vi "LIA Debugging Host.vi"() -> ()   [LabVIEW 2017]
uses:
  Program Files (x86)/National Instruments/LabVIEW 2017/examples/Lock-In Amplifier/lib/host/Public/pll settings.ctl
  Program Files (x86)/National Instruments/LabVIEW 2017/examples/Lock-In Amplifier/lib/host/Public/lock-in settings.ctl
  Program Files (x86)/National Instruments/LabVIEW 2017/examples/Lock-In Amplifier/lib/interface/Interface FPGA/LIA Host Interface FPGA.lvclass
  C:/Program Files (x86)/National Instruments/LabVIEW 2017/examples/Lock-In Amplifier/lib/interface/Interface/LIA Host Interface.lvclass
  Program Files (x86)/National Instruments/LabVIEW 2017/examples/Lock-In Amplifier/lib/host/Public/fpga type.ctl
  <vilib>/Analysis/4window.llb/windowTd.ctl
  <vilib>/measure/maspectr.llb/FFT Spectrum (Mag-Phase) for N Chan.vi
  Program Files (x86)/National Instruments/LabVIEW 2017/examples/Lock-In Amplifier/lib/interface/Interface FPGA/Properties/FpgaSession_GET.vi
  <vilib>/Utility/error.llb/Error Cluster From Error Code.vi
  <vilib>/rvi/errors/niLvFpgaAdjustHostInterfaceError.vi
  <vilib>/measure/maspectr.llb/FFT Power Spectrum and PSD for 1 Chan (CDB).vi
  <vilib>/measure/maspectr.llb/FFT Power Spectrum and PSD for N Chan.vi
  <vilib>/rvi/interface/nirviReadWriteControl/nirviReadWriteControl.xnode
  Program Files (x86)/National Instruments/LabVIEW 2017/examples/Lock-In Amplifier/lib/interface/Interface/LIA Host Interface.lvclass
  Program Files (x86)/National Instruments/LabVIEW 2017/examples/Lock-In Amplifier/lib/host/Lock-In Amplifier Example Host.lvlib
  Program Files (x86)/National Instruments/LabVIEW 2017/examples/Lock-In Amplifier/lib/shared/Lock-In Amplifier Example Shared.lvlib
  <vilib>/measure/NI_MAPro.lvlib
  NiFpgaLv.dll
  <vilib>/rvi/interface/Simulation/niFpgaSimulationCallBeginRW.vi
  <vilib>/Analysis/NI_AALPro.lvlib
  <vilib>/Analysis/NI_AALBase.lvlib
  <vilib>/ptbypt/NI_PtbyPt.lvlib
panel:
  in  "Tab Control 2":enum32{"Page 1", "Page 2"}(tab)
  in  "dpll.m 0":i8=-20
  in  "averaging lia":T1={"averaging mode"=enum."RMS averaging", "weighting mode"=enum."Exponential", "number of averages"=10}
  in  "restart averaging  lia":bool
  in  "lock-in.decimator0 0":enum16{"None", "CIC", "FIR", "4HB"}(ring)=enum."FIR"
  in  "lock-in.decimator1 0":enum16{"None", "FIR"}(ring)
  in  "averaging preview":T1={"averaging mode"=enum."RMS averaging", "weighting mode"=enum."Exponential", "number of averages"=10}
  in  "restart averaging preview":bool
  out "lock-in.max-min":dbl=1.9775797561733533e-07 caption="Deviation" format="%#_6p"
  out "lock-in.min":dbl=1.9775797561733533e-07 caption="Deviation" format="%#_6p"
  out "lock-in.max":dbl=1.9775797561733533e-07 caption="Deviation" format="%#_6p"
  in  "Tab Control 1":T2(tab)
  out "pll.vco output 0":fxp<+/-,48,0> format="%#.18g"
  out "lock-in.cic config 0":cluster{"factor":fxp<+,16,16>, "shift":i16}
  out "dpll.vco output 0":fxp<+/-,48,0> format="%#.18g"
  out "dpll.config 0":T3
  out "nco.frequency 0":fxp<+/-,48,0>=0.0010000000000012221 format="%#_48g"
  out "Waveform Graph 5":cluster{"f0":dbl, "df":dbl, "magnitude":dbl[]}(graph)
  out "Waveform Graph 2":cluster{"f0":dbl, "df":dbl, "magnitude":dbl[]}[](graph)
  out "Waveform Graph 3":dbl[][](graph)
  out "Waveform Graph 4":dbl[][](graph)
  out "Waveform Graph":cluster{"f0":dbl, "df":dbl, "magnitude":dbl[]}[](graph)
  in  "app.quit":bool
  in  "lock-in.record length 0":u32=2048 caption="Record Length"
  in  "app.tab 0":enum32{"Lock-In", "PLL"}(tab)
  in  "lock-in.decimation1 0":i32=2048 caption="Decimation 1"
  in  "lock-in.sampling rate":dbl=100000000.0 caption="Sampling Rate" format="%_10p"
  in  "lock-in.decimation0 0":i32=2048 caption="Decimation 0"
  in  "lock-in.source 0":enum16{"AI 0", "AI 1", "AI 2", "AI 3", "NCO 0"}(ring)=enum."AI 1" caption="Channel"
  in  "lock-in.carrier 0":T4(ring)=enum."DPLL 0" caption="Carrier Source"
  in  "lock-in.manual carrier 0":dbl=100000.0 caption="Carrier Frequency" format="%_10p"
  in  "pll.source 0":enum16{"AI 0", "AI 1", "AI 2", "AI 3"}(ring) caption="Source"
  in  "pll.q frequency 0":dbl=100000.0 caption="Q Frequency" format="%#_6p"
  in  "pll.reset 0":bool caption="PLL Reset"
  in  "rio device":tag="PXI1Slot8" caption="Resource"
  out "lock-in.deviation":dbl=1.9775797561733533e-07 caption="Deviation" format="%#_6p"
  out "lock-in.amplitude":dbl=8.221341747482856e-05 caption="lock-in.mean" format="%#_12p"
  out "Result":cluster{dbl, "standard deviation":dbl}(graph)
  # "NI Lock-In Amplifier Reference Example"
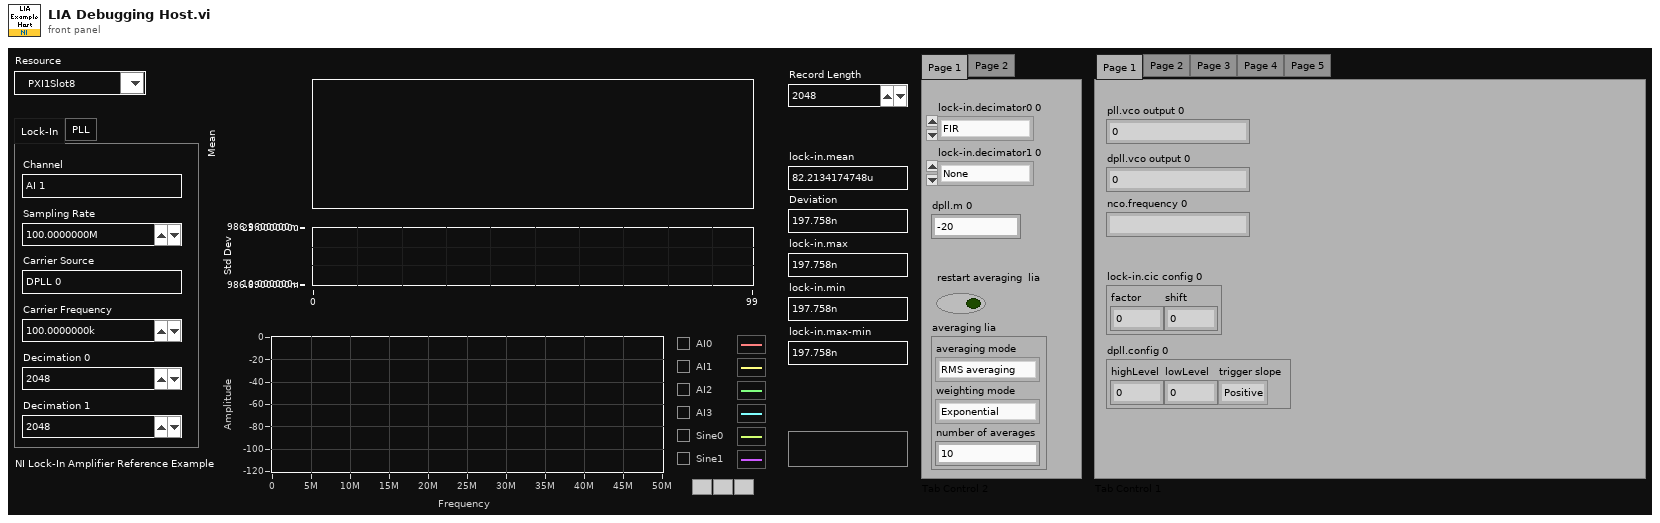
[diagram p1: front panel]
types:
  T1 = cluster{"averaging mode":enum16{"No averaging", "Vector averaging", "RMS averaging", "Peak hold"}, "weighting mode":enum16{"Linear", "Exponential"}, "number of averages":u32}
  T2 = enum32{"Page 1", "Page 2", "Page 3", "Page 4", "Page 5"}
  T3 = cluster{"highLevel":fxp<+/-,18,1>, "lowLevel":fxp<+/-,18,1>, "trigger slope":enum8{"Positive", "Negative"}}
  T4 = enum16{"Manual 0", "Manual 1", "Manual 2", "Manual 3", "PLL 0", "PLL 1", "DPLL 0", "DPLL 1"}
  T5 = typedef "Lock-In Amplifier Example Host.lvlib/lock-in settings.ctl" = cluster{"decimation":i32, "source":i32, "carrier source":i32, "carrier":dbl}
  T6 = typedef "Lock-In Amplifier Example Host.lvlib/pll settings.ctl" = cluster{"source":i32, "q frequency":dbl}
  T7 = typedef "NI_AALPro.lvlib/windowTd.ctl" = u32
  T8 = cluster{"dB On (F)":bool, "unwrap phase (F)":bool, "convert to degree (F)":bool}
  T9 = typedef "Lock-In Amplifier Example Host.lvlib/fpga type.ctl" = refnum<k20>
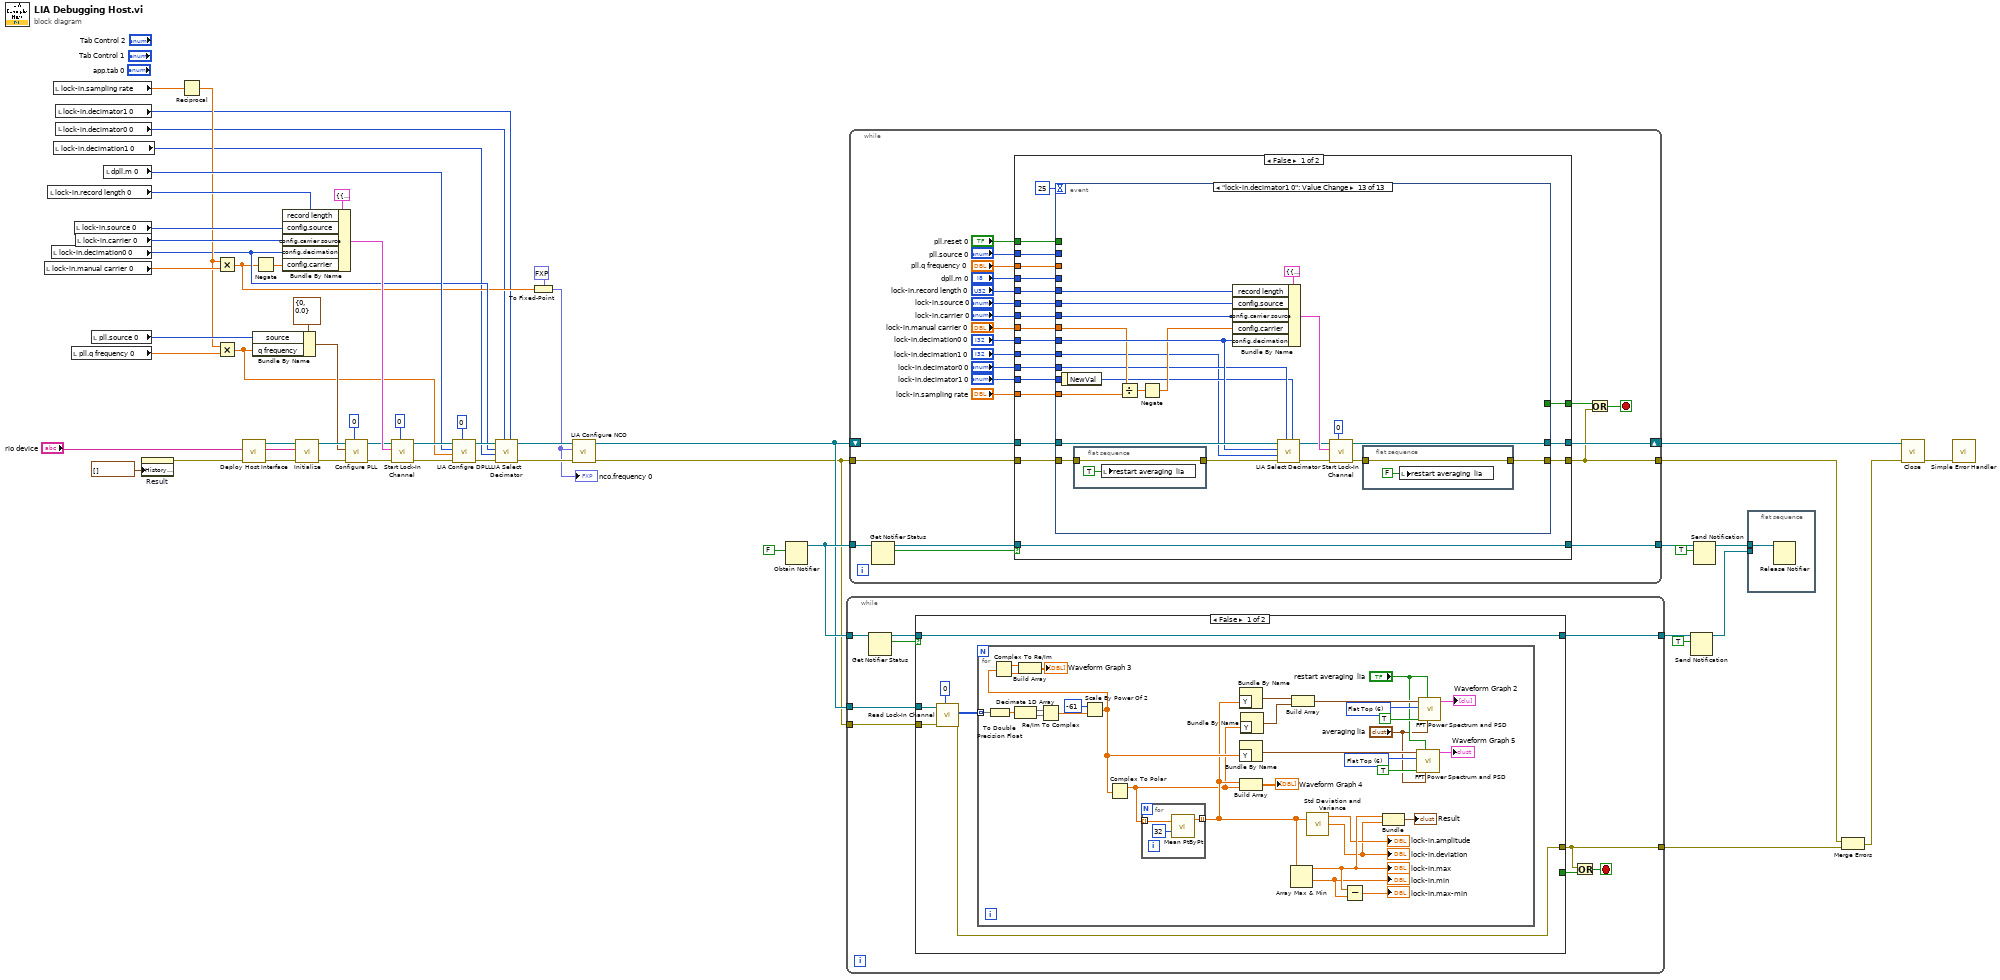
[diagram p0: block diagram]
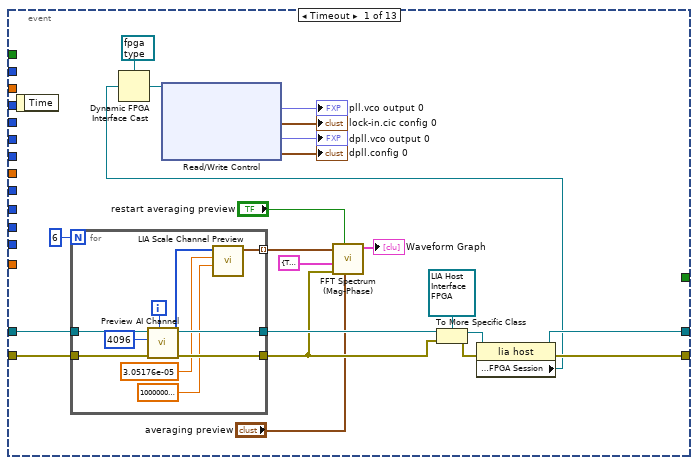
[diagram p2: hidden frame]
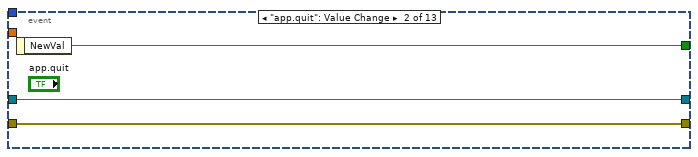
[diagram p3: hidden frame]
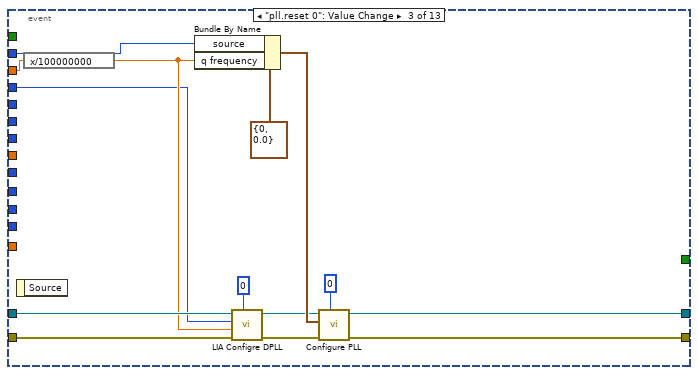
[diagram p4: hidden frame]
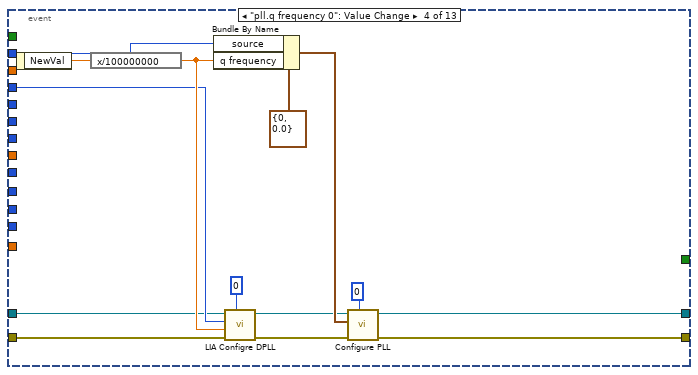
[diagram p5: hidden frame]
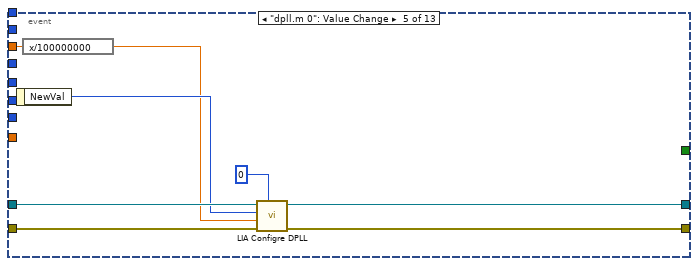
[diagram p6: hidden frame]
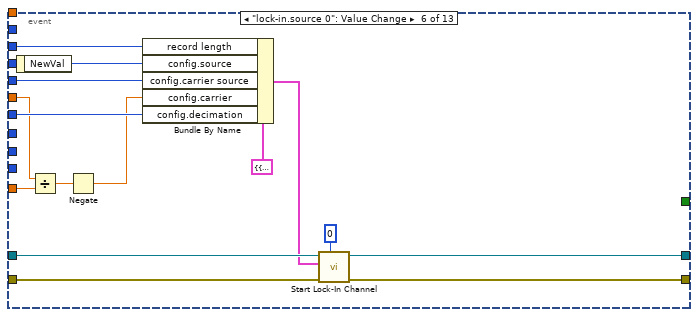
[diagram p7: hidden frame]
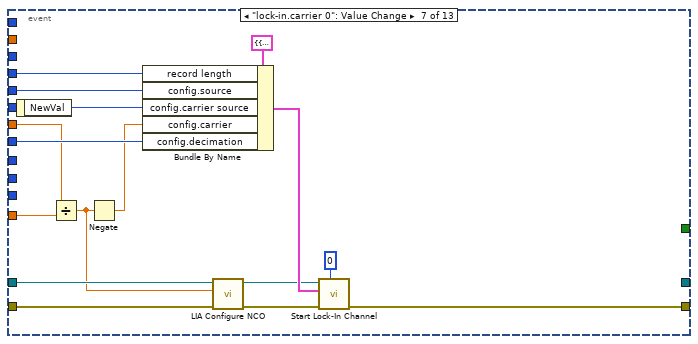
[diagram p8: hidden frame]
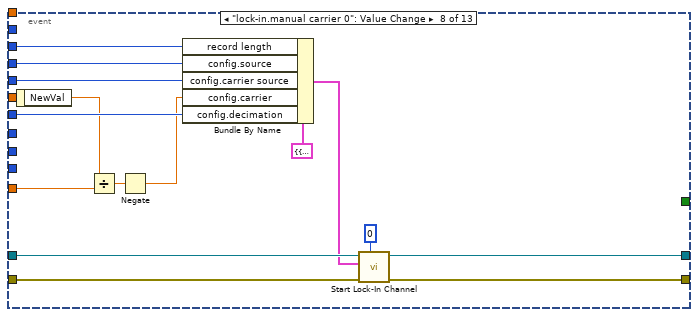
[diagram p9: hidden frame]
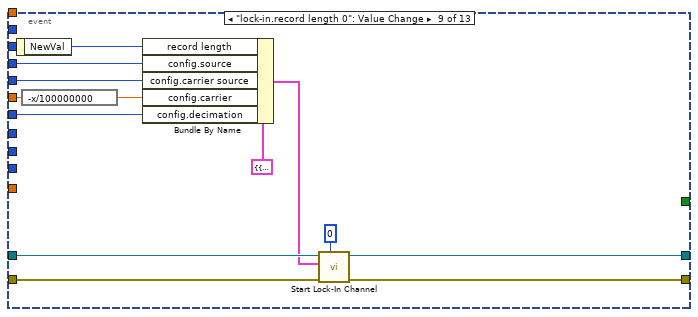
[diagram p10: hidden frame]
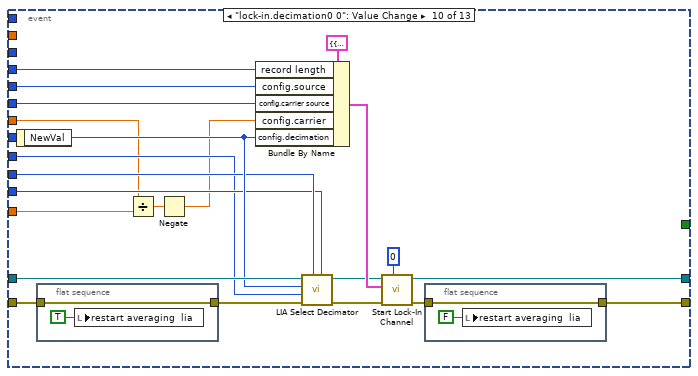
[diagram p11: hidden frame]
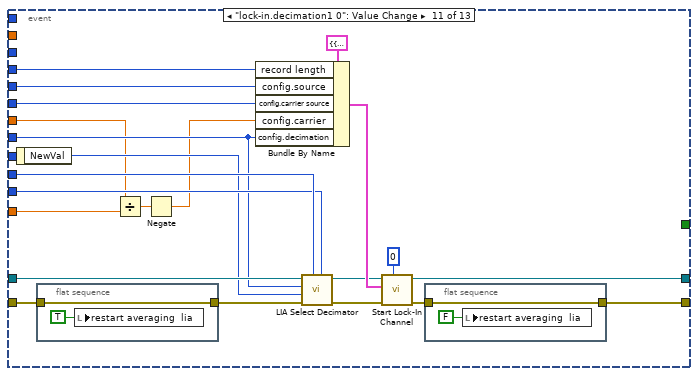
[diagram p12: hidden frame]
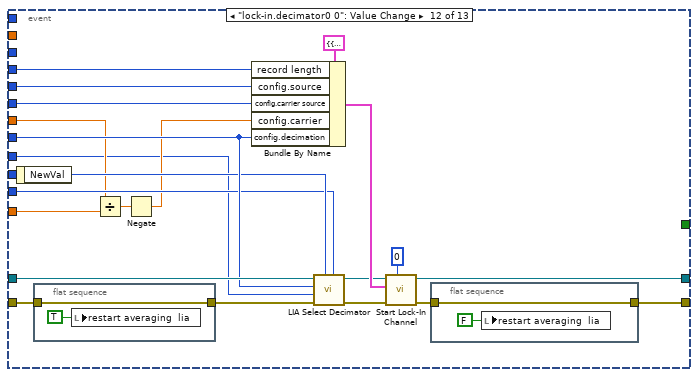
[diagram p13: hidden frame]
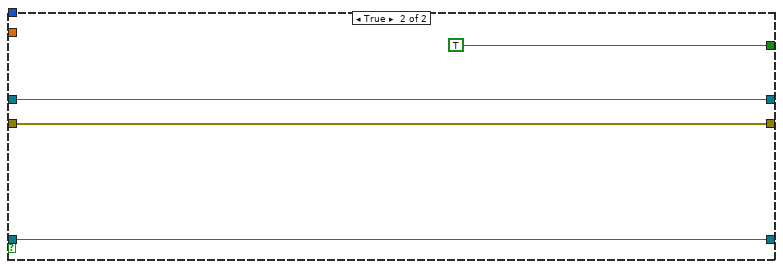
[diagram p14: hidden frame]
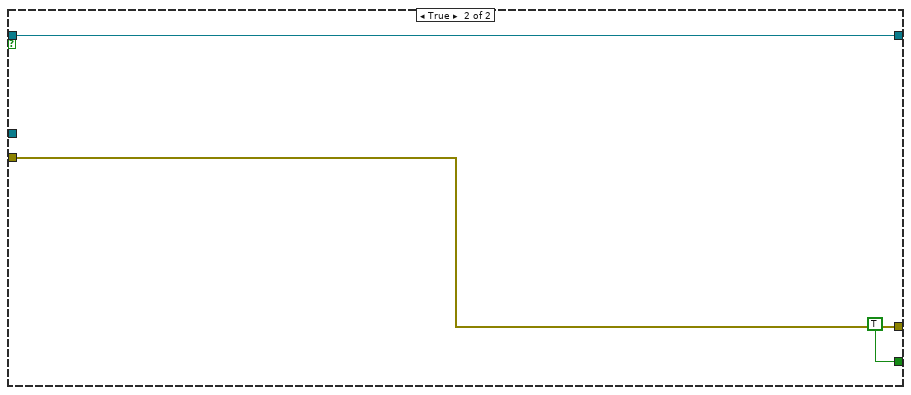
[diagram p15: hidden frame]
diagram:
  n1 = local read "lock-in.manual carrier 0"() -> (w51:dbl)
  n2 = local read "lock-in.record length 0"() -> (w32:u32)
  n3 = local read "lock-in.decimation0 0"() -> (w7:i32)
  n4 = local read "lock-in.sampling rate"() -> (w8:dbl)
  n5 = local read "lock-in.decimation1 0"() -> (w1:i32)
  n6 = local read "lock-in.decimator1 0"() -> (w2:enum16{"None", "FIR"})
  n7 = local read "lock-in.decimator0 0"() -> (w3:enum16{"None", "CIC", "FIR", "4HB"})
  n8 = local read "pll.q frequency 0"() -> (w52:dbl)
  n9 = local read "lock-in.source 0"() -> (w56:enum16{"AI 0", "AI 1", "AI 2", "AI 3", "NCO 0"})
  n10 = local read "lock-in.carrier 0"() -> (w55:T4)
  n11 = local read "pll.source 0"() -> (w53:enum16{"AI 0", "AI 1", "AI 2", "AI 3"})
  n12 = local read "dpll.m 0"() -> (w18:i8)
  n13 = property on="Result" class="WFChart (strict)"("History Data"=cluster{dbl, "standard deviation":dbl}[] []) -> (error out=w27:errorcluster)  [unwired: 2 in, 1 out]
  n14 = Reciprocal(x=w8) -> (1/x=w13:dbl)
  n15 = Multiply(x=w13, y=w51) -> (x*y=w6:dbl)
  n16 = Multiply(x=w13, y=w52) -> (x*y=w11:dbl)
  n17 = call "Deploy Host Interface.vi"("error in"=w27, "resource"="rio device") -> ("error out"=w28:errorcluster, "resource out"=w29:string, "lia host interface"=w30:refnum<class "LIA Host Interface.lvclass">)  [unwired: 7 in]
  n18 = Bundle By Name(cluster=T6 {"source"=0, "q frequency"=0.0} ("config"), "source"=w53, "q frequency"=w11) -> (w12:T6)
  n19 = Negate(x=w6) -> (-x=w4:dbl)
  n20 = Bundle By Name(cluster=cluster{"config":T5, "record length":u32} {"config"={"decimation"=0, "source"=0, "carrier source"=0, "carrier"=0.0}, "record length"=0} ("config"), "record length"=w32, "config.source"=w56, "config.carrier source"=w55, "config.decimation"=w7, "config.carrier"=w4) -> (w33:cluster{"config":T5, "record length":u32})
  n21 = call-dynamic "Initialize.vi"("error in"=w28, "resource"=w29, "lia host in"=w30) -> ("error out"=w37:errorcluster, "lia host out"=w38:refnum<class "LIA Host Interface.lvclass">)  [unwired: 7 in]
  n22 = call-dynamic "Configure PLL.vi"("instance"=0 ("index"), "error in"=w37, "config"=w12, "lia host in"=w38) -> ("error out"=w26:errorcluster, "lia host out"=w25:refnum<class "LIA Host Interface.lvclass">)  [unwired: 6 in]
  n23 = call-dynamic "Start Lock-In Channel.vi"("instance"=0 ("index"), "error in"=w26, "config"=w33, "lia host in"=w25) -> ("error out"=w23:errorcluster, "lia host out"=w21:refnum<class "LIA Host Interface.lvclass">)  [unwired: 6 in]
  n24 = call "LIA Configre DPLL.vi"("dpll.channel 0"=0, "error in (no error)"=w23, "dpll.q 0"=w11, "dpll.m 0"=w18, "LIA Host Interface in"=w21) -> ("error out"=w19:errorcluster, "LIA Host Interface Out"=w20:refnum<class "LIA Host Interface.lvclass">)  [unwired: 5 in]
  n25 = call "LIA Select Decimator.vi"("lock-in.decimator1 0"=w2, "lock-in.decimator0 0"=w3, "error in (no error)"=w19, "lock-in.decimation1 0"=w1, "lock-in.decimation0 0"=w7, "LIA Host Interface in"=w20) -> ("error out"=w16:errorcluster, "LIA Host Interface out"=w17:refnum<class "LIA Host Interface.lvclass">)  [unwired: 4 in]
  n26 = To Fixed-Point(fixed-point type=fxp<+/-,48,0> 0.0 ("nco.frequency 0"), number=w6) -> (fixed-point=w10:fxp<+/-,48,0>)
  "nco.frequency 0" <- w10
  n27 = call "LIA Configure NCO.vi"("error in (no error)"=w16, "nco.frequency 0"=w10, "LIA Host Interface in"=w17) -> ("error out"=w14:errorcluster, "LIA Host Interface out"=w15:refnum<class "LIA Host Interface.lvclass">)  [unwired: 7 in]
  n28 = Obtain Notifier(notification data type=FALSE) -> (notifier out=w48:refnum<notifier>)  [unwired: 3 in, 2 out]
  n29 = while {
    tunnel: w48 -> [w65]
    tunnel: w15 -> [w62]
    tunnel: w14 -> [w61]
    tunnel: [w60] -> w41
    tunnel: [w57] -> w44
    stop <- w59 stop-if-true
    n30 = Get Notifier Status(notifier=w65) -> (notifier out=w63:refnum<notifier>, current notification=w64:bool)  [unwired: 1 in, 3 out]
    n31 = case shown="False" w64 {
      tunnel: [w68 w108] -> w57
      tunnel: w63 -> [w68 w108]
      tunnel: w62 -> [w71 _]
      tunnel: w61 -> [w70 w107]
      tunnel: [w66 w107] -> w60
      tunnel: [_ TRUE] -> w58
      frame False {
        n32 = call-dynamic "Read Lock-In Channel.vi"("instance"=0 ("index"), "error in"=w70, "lia host in"=w71) -> ("error out"=w66:errorcluster, "unscaled data"=w67:i64[][])  [unwired: 6 in, 1 out]
        n33 = for {
          tunnel: w67 -> [w98] mode=indexing
          w78 = T7 6 items=["Rectangle"=0, "Hanning"=1, "Hamming"=2, "Blackman-Harris"=3, "Exact Blackman"=4, "Blackman"=5, "Flat Top"=6, "4 Term B-Harris "=7, "7 Term B-Harris"=8, "Low Sidelobe"=9, "Blackman Nuttall"=11, "Triangle"=30, "Bartlett-Hanning"=31, "Bohman"=32, "Parzen"=33, "Welch"=34, "Kaiser"=60, "Dolph-Chebyshev"=61, "Gaussian"=62] ("window")
          w102 = T7 6 items=["Rectangle"=0, "Hanning"=1, "Hamming"=2, "Blackman-Harris"=3, "Exact Blackman"=4, "Blackman"=5, "Flat Top"=6, "4 Term B-Harris "=7, "7 Term B-Harris"=8, "Low Sidelobe"=9, "Blackman Nuttall"=11, "Triangle"=30, "Bartlett-Hanning"=31, "Bohman"=32, "Parzen"=33, "Welch"=34, "Kaiser"=60, "Dolph-Chebyshev"=61, "Gaussian"=62] ("window")
          n34 = To Double Precision Float(number=w98) -> (double precision float=w100:dbl[])
          n35 = Decimate 1D Array(w100) -> (w89:dbl[], w87:dbl[])
          n36 = Re/Im To Complex(1:w87, 2:w89) -> (0:w99:cdb[])
          n37 = Scale By Power Of 2(n=i16 -61, x=w99) -> (x*2^n=w77:cdb[])
          n38 = Complex To Re/Im(x + iy=w77) -> (x=w86:dbl[], y=w85:dbl[])
          n39 = Build Array(w86, w85) -> (→"Waveform Graph 3":dbl[][])
          n40 = Complex To Polar(r * e^(i*theta)=w77) -> (r=w74:dbl[])  [unwired: 1 out]
          n41 = for {
            tunnel: w74 -> [w105] mode=indexing
            tunnel: [w104] -> w75 mode=indexing
            n42 = call <vilib>:"Mean PtByPt.vi"("x"=w105, "sample length"=32) -> ("mean"=w104:dbl)  [unwired: 2 in, 1 out]
          }
          n43 = Bundle By Name("Y"=w75) -> (w83:waveform(dbl))  [unwired: 1 in]
          n44 = Bundle By Name("Y"=w77) -> (w76:waveform(cdb))  [unwired: 1 in]
          n45 = Build Array(w75, w74) -> (→"Waveform Graph 4":dbl[][])
          n46 = Bundle By Name("Y"=w74) -> (w82:waveform(dbl))  [unwired: 1 in]
          n47 = Array Max & Min(array=w75) -> (max value=w93:dbl, min value=w91:dbl)  [unwired: 2 out]
          "lock-in.max" <- w93
          "lock-in.min" <- w91
          n48 = Build Array(w83, w82) -> (w81:waveform(dbl)[])
          n49 = call <vilib>:"Std Deviation and Variance.vi"("X"=w75) -> ("mean"=→"lock-in.amplitude":dbl, "standard deviation"=w90:dbl)  [unwired: 1 in, 1 out]
          "lock-in.deviation" <- w90
          n50 = Subtract(x=w93, y=w91) -> (x-y=→"lock-in.max-min":dbl)
          n51 = Bundle(w93, "standard deviation"=w90) -> (→"Result":cluster{dbl, "standard deviation":dbl})  [unwired: 1 in]
          n52 = call-poly <vilib>:"FFT Power Spectrum and PSD.vi"("averaging parameters"="averaging lia", "restart averaging (F)"="restart averaging  lia", "dB On (F)"=TRUE, "window"=w78, "time signal"=w76) -> ("Power Spectrum / PSD"=→"Waveform Graph 5":cluster{"f0":dbl, "df":dbl, "magnitude":dbl[]})  [unwired: 3 in, 3 out]
          n53 = call-poly <vilib>:"FFT Power Spectrum and PSD.vi"("averaging parameters"="averaging lia", "restart averaging (F)"="restart averaging  lia", "dB On (F)"=TRUE, "window"=w102, "time signals"=w81) -> ("Power Spectrum / PSD"=→"Waveform Graph 2":cluster{"f0":dbl, "df":dbl, "magnitude":dbl[]}[])  [unwired: 3 in, 3 out]
        }
      }
      frame True {
      }
    }
    n54 = Or(x=w60, y=w58) -> (x .or. y?=w59:bool)
  }
  n55 = while {
    tunnel: w14 -> [w131]
    shift-right: [w123] -> w50
    shift-left: w15 -> [w130]
    tunnel: [w119] -> w40
    tunnel: w48 -> [w122]
    tunnel: [w117] -> w47
    stop <- w129 stop-if-true
    n56 = Get Notifier Status(notifier=w122) -> (notifier out=w121:refnum<notifier>, current notification=w120:bool)  [unwired: 1 in, 3 out]
    n57 = case shown="False" w120 {
      tunnel: w131 -> [w151 w388]
      tunnel: w130 -> [w150 w389]
      tunnel: [w149 w388] -> w119
      tunnel: "lock-in.manual carrier 0" -> [w147 _]
      tunnel: "lock-in.decimation0 0" -> [w146 _]
      tunnel: "lock-in.source 0" -> [w145 _]
      tunnel: "lock-in.carrier 0" -> [w144 _]
      tunnel: "pll.source 0" -> [w143 _]
      tunnel: "pll.q frequency 0" -> [w142 _]
      tunnel: [w141 w389] -> w123
      tunnel: w121 -> [w139 w386]
      tunnel: [w140 TRUE] -> w118
      tunnel: [w139 w386] -> w117
      tunnel: "lock-in.record length 0" -> [w138 _]
      tunnel: "dpll.m 0" -> [w137 _]
      tunnel: "lock-in.decimator0 0" -> [w136 _]
      tunnel: "lock-in.sampling rate" -> [w135 _]
      tunnel: "pll.reset 0" -> [w134 _]
      tunnel: "lock-in.decimator1 0" -> [w133 _]
      tunnel: "lock-in.decimation1 0" -> [w132 _]
      frame False {
        n58 = event shown="[12] \"lock-in.decimator1 0\": Value Change" {
          selector: _ -> [_ _ _ _ _ _ _ _ _ _ _ _ _]
          dyn-events: _ -> [_ _ _ _ _ _ _ _ _ _ _ _ _]
          timeout: 25 -> [_ _ _ _ _ _ _ _ _ _ _ _ _]
          tunnel: w151 -> [w172 w185 w190 w201 w217 w235 w243 w266 w277 w292 w319 w343 w369]
          tunnel: w150 -> [w173 w186 w192 w202 w222 w233 w245 w264 w275 w294 w320 w346 w372]
          tunnel: [w166 w185 w200 w210 w215 w234 w252 w265 w276 w289 w316 w342 w368] -> w149
          tunnel: w145 -> [_ _ _ _ _ _ w246 w258 w269 w300 w326 w352 w378]
          tunnel: w144 -> [_ _ _ _ _ w237 _ w268 w280 w303 w329 w355 w381]
          tunnel: w147 -> [_ _ _ _ w219 w225 w240 _ w279 w283 w310 w336 w364]
          tunnel: w146 -> [_ _ _ _ _ w236 w253 w267 w278 _ w312 w345 w371]
          tunnel: w143 -> [_ _ w197 w213 _ _ _ _ _ _ _ _ _]
          tunnel: w142 -> [_ _ w194 _ _ _ _ _ _ _ _ _ _]
          tunnel: [w167 w186 w195 w211 w216 w232 _ w263 w274 w302 w328 w354 w380] -> w141
          tunnel: [_ w184 _ _ _ _ _ _ _ _ _ _ _] -> w140
          tunnel: w138 -> [_ _ _ _ _ w229 w249 w260 _ w298 w324 w350 w376]
          tunnel: w137 -> [_ _ w187 w205 _ _ _ _ _ _ _ _ _]
          tunnel: w136 -> [_ _ _ _ _ _ _ _ _ w288 w315 _ w362]
          tunnel: w135 -> [_ _ _ _ _ w224 w241 w255 _ w284 w309 w337 w365]
          tunnel: w134 -> [_ _ _ _ _ _ _ _ _ _ _ _ _]
          tunnel: w133 -> [_ _ _ _ _ _ _ _ _ w287 w314 w339 _]
          tunnel: w132 -> [_ _ _ _ _ _ _ _ _ w286 _ w334 w360]
          event Timeout {
            n59 = event-data() -> ()  [unwired: 1 in, 1 out]
            n60 = for {
              N: 6 -> [_]
              tunnel: w173 -> [w183]
              tunnel: [w181] -> w168
              tunnel: w172 -> [w182]
              tunnel: [w178] -> w156
              tunnel: [w176] -> w154 mode=indexing
              i -> [w179]
              n61 = call-dynamic "Preview AI Channel.vi"("instance"=w179, "error in"=w182, "samples"=u32 4096, "lia host in"=w183) -> ("error out"=w178:errorcluster, "samples"=w177:i16[], "lia host out"=w181:refnum<class "LIA Host Interface.lvclass">)  [unwired: 5 in]
              n62 = call "LIA Scale Channel Preview.vi"("sample rate"=100000000.0, "scaling factor"=3.05176e-05, "ai data"=w177) -> ("Waveform"=w176:waveform(dbl))  [unwired: 8 in]
            }
            n63 = call-poly <vilib>:"FFT Spectrum (Mag-Phase).vi"("averaging parameters"="averaging preview", "restart averaging (F)"="restart averaging preview", "error in (no error)"=w156, "view"=T8 {"dB On (F)"=TRUE, "unwrap phase (F)"=FALSE, "convert to degree (F)"=FALSE}, "time signals"=w154) -> ("magnitudes"=→"Waveform Graph":cluster{"f0":dbl, "df":dbl, "magnitude":dbl[]}[])  [unwired: 2 in, 4 out]
            n64 = To More Specific Class(target class=refnum<class "LIA Host Interface FPGA.lvclass"> refnum ("lia host"), reference=w168, error in=w156) -> (specific class reference=w170:refnum<class "LIA Host Interface FPGA.lvclass">, error out=w158:errorcluster)
            n65 = property class="lia host"(reference=w170, error in=w158) -> (reference out=w167:refnum<class "LIA Host Interface FPGA.lvclass">, error out=w166:errorcluster, "Properties:FPGA Session"=w165:refnum<k20>)
            n66 = Dynamic FPGA Interface Cast(Session In=T9 refnum ("fpga type"), Type=w165) -> (Session Out=w163:T9)
            n67 = xnode "Read/Write Control"("FPGA VI Reference In"=w163) -> ("pll.vco output 0"=→"pll.vco output 0":fxp<+/-,48,0>, "lock-in.cic config 0"=→"lock-in.cic config 0":cluster{"factor":fxp<+,16,16>, "shift":i16}, "dpll.vco output 0"=→"dpll.vco output 0":fxp<+/-,48,0>, "dpll.config 0"=→"dpll.config 0":T3)  [unwired: 1 in, 2 out]
          }
          event "app.quit": Value Change {
            n68 = event-data() -> ("NewVal"=w184:bool)  [unwired: 1 in]
          }
          event "pll.reset 0": Value Change {
            n69 = event-data() -> ()  [unwired: 1 in, 1 out]
            n70 = expression code="x/100000000"(w194) -> (w188:dbl)
            n71 = Bundle By Name(cluster=T6 {"source"=0, "q frequency"=0.0} ("config"), "source"=w197, "q frequency"=w188) -> (w196:T6)
            n72 = call "LIA Configre DPLL.vi"("dpll.channel 0"=0, "error in (no error)"=w190, "dpll.q 0"=w188, "dpll.m 0"=w187, "LIA Host Interface in"=w192) -> ("error out"=w189:errorcluster, "LIA Host Interface Out"=w191:refnum<class "LIA Host Interface.lvclass">)  [unwired: 5 in]
            n73 = call-dynamic "Configure PLL.vi"("instance"=0 ("index"), "error in"=w189, "config"=w196, "lia host in"=w191) -> ("error out"=w200:errorcluster, "lia host out"=w195:refnum<class "LIA Host Interface.lvclass">)  [unwired: 6 in]
          }
          event "pll.q frequency 0": Value Change {
            n74 = event-data() -> ("NewVal"=w212:dbl)  [unwired: 1 in]
            n75 = expression code="x/100000000"(w212) -> (w206:dbl)
            n76 = Bundle By Name(cluster=T6 {"source"=0, "q frequency"=0.0} ("config"), "source"=w213, "q frequency"=w206) -> (w209:T6)
            n77 = call "LIA Configre DPLL.vi"("dpll.channel 0"=0, "error in (no error)"=w201, "dpll.q 0"=w206, "dpll.m 0"=w205, "LIA Host Interface in"=w202) -> ("error out"=w203:errorcluster, "LIA Host Interface Out"=w204:refnum<class "LIA Host Interface.lvclass">)  [unwired: 5 in]
            n78 = call-dynamic "Configure PLL.vi"("instance"=0, "error in"=w203, "config"=w209, "lia host in"=w204) -> ("error out"=w210:errorcluster, "lia host out"=w211:refnum<class "LIA Host Interface.lvclass">)  [unwired: 6 in]
          }
          event "dpll.m 0": Value Change {
            n79 = event-data() -> ("NewVal"=w220:i8)  [unwired: 1 in]
            n80 = expression code="x/100000000"(w219) -> (w218:dbl)
            n81 = call "LIA Configre DPLL.vi"("dpll.channel 0"=0, "error in (no error)"=w217, "dpll.q 0"=w218, "dpll.m 0"=w220, "LIA Host Interface in"=w222) -> ("error out"=w215:errorcluster, "LIA Host Interface Out"=w216:refnum<class "LIA Host Interface.lvclass">)  [unwired: 5 in]
          }
          event "lock-in.source 0": Value Change {
            n82 = event-data() -> ("NewVal"=w227:enum16{"AI 0", "AI 1", "AI 2", "AI 3", "NCO 0"})  [unwired: 1 in]
            n83 = Divide(x=w225, y=w224) -> (x/y=w226:dbl)
            n84 = Negate(x=w226) -> (-x=w223:dbl)
            n85 = Bundle By Name(cluster=cluster{"config":T5, "record length":u32} {"config"={"decimation"=0, "source"=0, "carrier source"=0, "carrier"=0.0}, "record length"=0} ("config"), "record length"=w229, "config.source"=w227, "config.carrier source"=w237, "config.carrier"=w223, "config.decimation"=w236) -> (w228:cluster{"config":T5, "record length":u32})
            n86 = call-dynamic "Start Lock-In Channel.vi"("instance"=0 ("index"), "error in"=w235, "config"=w228, "lia host in"=w233) -> ("error out"=w234:errorcluster, "lia host out"=w232:refnum<class "LIA Host Interface.lvclass">)  [unwired: 6 in]
          }
          event "lock-in.carrier 0": Value Change {
            n87 = event-data() -> ("NewVal"=w247:T4)  [unwired: 1 in]
            n88 = Divide(x=w240, y=w241) -> (x/y=w238:dbl)
            n89 = Negate(x=w238) -> (-x=w239:dbl)
            n90 = Bundle By Name(cluster=cluster{"config":T5, "record length":u32} {"config"={"decimation"=0, "source"=0, "carrier source"=0, "carrier"=0.0}, "record length"=0} ("config"), "record length"=w249, "config.source"=w246, "config.carrier source"=w247, "config.carrier"=w239, "config.decimation"=w253) -> (w248:cluster{"config":T5, "record length":u32})
            n91 = call "LIA Configure NCO.vi"("error in (no error)"=w243, "nco.frequency 0"=w238, "LIA Host Interface in"=w245) -> ("error out"=w242:errorcluster, "LIA Host Interface out"=w244:refnum<class "LIA Host Interface.lvclass">)  [unwired: 7 in]
            n92 = call-dynamic "Start Lock-In Channel.vi"("instance"=0 ("index"), "error in"=w242, "config"=w248, "lia host in"=w244) -> ("error out"=w252:errorcluster)  [unwired: 6 in, 1 out]
          }
          event "lock-in.manual carrier 0": Value Change {
            n93 = event-data() -> ("NewVal"=w256:dbl)  [unwired: 1 in]
            n94 = Divide(x=w256, y=w255) -> (x/y=w257:dbl)
            n95 = Negate(x=w257) -> (-x=w254:dbl)
            n96 = Bundle By Name(cluster=cluster{"config":T5, "record length":u32} {"config"={"decimation"=0, "source"=0, "carrier source"=0, "carrier"=0.0}, "record length"=0} ("config"), "record length"=w260, "config.source"=w258, "config.carrier source"=w268, "config.carrier"=w254, "config.decimation"=w267) -> (w259:cluster{"config":T5, "record length":u32})
            n97 = call-dynamic "Start Lock-In Channel.vi"("instance"=0 ("index"), "error in"=w266, "config"=w259, "lia host in"=w264) -> ("error out"=w265:errorcluster, "lia host out"=w263:refnum<class "LIA Host Interface.lvclass">)  [unwired: 6 in]
          }
          event "lock-in.record length 0": Value Change {
            n98 = event-data() -> ("NewVal"=w270:u32)  [unwired: 1 in]
            n99 = expression code="-x/100000000"(w279) -> (w281:dbl)
            n100 = Bundle By Name(cluster=cluster{"config":T5, "record length":u32} {"config"={"decimation"=0, "source"=0, "carrier source"=0, "carrier"=0.0}, "record length"=0} ("config"), "record length"=w270, "config.source"=w269, "config.carrier source"=w280, "config.carrier"=w281, "config.decimation"=w278) -> (w271:cluster{"config":T5, "record length":u32})
            n101 = call-dynamic "Start Lock-In Channel.vi"("instance"=0 ("index"), "error in"=w277, "config"=w271, "lia host in"=w275) -> ("error out"=w276:errorcluster, "lia host out"=w274:refnum<class "LIA Host Interface.lvclass">)  [unwired: 6 in]
          }
          event "lock-in.decimation0 0": Value Change {
            n102 = event-data() -> ("NewVal"=w293:i32)  [unwired: 1 in]
            n103 = flat-sequence {
              tunnel: [w306] -> w291
              tunnel: w292 -> [w306]
              frame #0 {
                n104 = local write "restart averaging  lia"(TRUE ("restart averaging  lia")) -> ()
              }
            }
            n105 = Divide(x=w283, y=w284) -> (x/y=w285:dbl)
            n106 = Negate(x=w285) -> (-x=w282:dbl)
            n107 = Bundle By Name(cluster=cluster{"config":T5, "record length":u32} {"config"={"decimation"=0, "source"=0, "carrier source"=0, "carrier"=0.0}, "record length"=0} ("config"), "record length"=w298, "config.source"=w300, "config.carrier source"=w303, "config.carrier"=w282, "config.decimation"=w293) -> (w297:cluster{"config":T5, "record length":u32})
            n108 = call "LIA Select Decimator.vi"("lock-in.decimator1 0"=w287, "lock-in.decimator0 0"=w288, "error in (no error)"=w291, "lock-in.decimation1 0"=w286, "lock-in.decimation0 0"=w293, "LIA Host Interface in"=w294) -> ("error out"=w295:errorcluster, "LIA Host Interface out"=w296:refnum<class "LIA Host Interface.lvclass">)  [unwired: 4 in]
            n109 = call-dynamic "Start Lock-In Channel.vi"("instance"=0 ("index"), "error in"=w295, "config"=w297, "lia host in"=w296) -> ("error out"=w290:errorcluster, "lia host out"=w302:refnum<class "LIA Host Interface.lvclass">)  [unwired: 6 in]
            n110 = flat-sequence {
              tunnel: [w304] -> w289
              tunnel: w290 -> [w304]
              frame #0 {
                n111 = local write "restart averaging  lia"(FALSE ("restart averaging  lia")) -> ()
              }
            }
          }
          event "lock-in.decimation1 0": Value Change {
            n112 = event-data() -> ("NewVal"=w313:i32)  [unwired: 1 in]
            n113 = flat-sequence {
              tunnel: [w332] -> w318
              tunnel: w319 -> [w332]
              frame #0 {
                n114 = local write "restart averaging  lia"(TRUE ("restart averaging  lia")) -> ()
              }
            }
            n115 = Divide(x=w310, y=w309) -> (x/y=w311:dbl)
            n116 = Negate(x=w311) -> (-x=w308:dbl)
            n117 = Bundle By Name(cluster=cluster{"config":T5, "record length":u32} {"config"={"decimation"=0, "source"=0, "carrier source"=0, "carrier"=0.0}, "record length"=0} ("config"), "record length"=w324, "config.source"=w326, "config.carrier source"=w329, "config.carrier"=w308, "config.decimation"=w312) -> (w323:cluster{"config":T5, "record length":u32})
            n118 = call "LIA Select Decimator.vi"("lock-in.decimator1 0"=w314, "lock-in.decimator0 0"=w315, "error in (no error)"=w318, "lock-in.decimation1 0"=w313, "lock-in.decimation0 0"=w312, "LIA Host Interface in"=w320) -> ("error out"=w321:errorcluster, "LIA Host Interface out"=w322:refnum<class "LIA Host Interface.lvclass">)  [unwired: 4 in]
            n119 = call-dynamic "Start Lock-In Channel.vi"("instance"=0 ("index"), "error in"=w321, "config"=w323, "lia host in"=w322) -> ("error out"=w317:errorcluster, "lia host out"=w328:refnum<class "LIA Host Interface.lvclass">)  [unwired: 6 in]
            n120 = flat-sequence {
              tunnel: [w330] -> w316
              tunnel: w317 -> [w330]
              frame #0 {
                n121 = local write "restart averaging  lia"(FALSE ("restart averaging  lia")) -> ()
              }
            }
          }
          event "lock-in.decimator0 0": Value Change {
            n122 = event-data() -> ("NewVal"=w340:enum16{"None", "CIC", "FIR", "4HB"})  [unwired: 1 in]
            n123 = flat-sequence {
              tunnel: [w358] -> w344
              tunnel: w343 -> [w358]
              frame #0 {
                n124 = local write "restart averaging  lia"(TRUE ("restart averaging  lia")) -> ()
              }
            }
            n125 = Divide(x=w336, y=w337) -> (x/y=w338:dbl)
            n126 = Negate(x=w338) -> (-x=w335:dbl)
            n127 = Bundle By Name(cluster=cluster{"config":T5, "record length":u32} {"config"={"decimation"=0, "source"=0, "carrier source"=0, "carrier"=0.0}, "record length"=0} ("config"), "record length"=w350, "config.source"=w352, "config.carrier source"=w355, "config.carrier"=w335, "config.decimation"=w345) -> (w349:cluster{"config":T5, "record length":u32})
            n128 = call "LIA Select Decimator.vi"("lock-in.decimator1 0"=w339, "lock-in.decimator0 0"=w340, "error in (no error)"=w344, "lock-in.decimation1 0"=w334, "lock-in.decimation0 0"=w345, "LIA Host Interface in"=w346) -> ("error out"=w347:errorcluster, "LIA Host Interface out"=w348:refnum<class "LIA Host Interface.lvclass">)  [unwired: 4 in]
            n129 = call-dynamic "Start Lock-In Channel.vi"("instance"=0 ("index"), "error in"=w347, "config"=w349, "lia host in"=w348) -> ("error out"=w341:errorcluster, "lia host out"=w354:refnum<class "LIA Host Interface.lvclass">)  [unwired: 6 in]
            n130 = flat-sequence {
              tunnel: [w356] -> w342
              tunnel: w341 -> [w356]
              frame #0 {
                n131 = local write "restart averaging  lia"(FALSE ("restart averaging  lia")) -> ()
              }
            }
          }
          event "lock-in.decimator1 0": Value Change {
            n132 = event-data() -> ("NewVal"=w361:enum16{"None", "FIR"})  [unwired: 1 in]
            n133 = flat-sequence {
              tunnel: [w384] -> w370
              tunnel: w369 -> [w384]
              frame #0 {
                n134 = local write "restart averaging  lia"(TRUE ("restart averaging  lia")) -> ()
              }
            }
            n135 = Divide(x=w364, y=w365) -> (x/y=w366:dbl)
            n136 = Negate(x=w366) -> (-x=w363:dbl)
            n137 = Bundle By Name(cluster=cluster{"config":T5, "record length":u32} {"config"={"decimation"=0, "source"=0, "carrier source"=0, "carrier"=0.0}, "record length"=0} ("config"), "record length"=w376, "config.source"=w378, "config.carrier source"=w381, "config.carrier"=w363, "config.decimation"=w371) -> (w375:cluster{"config":T5, "record length":u32})
            n138 = call "LIA Select Decimator.vi"("lock-in.decimator1 0"=w361, "lock-in.decimator0 0"=w362, "error in (no error)"=w370, "lock-in.decimation1 0"=w360, "lock-in.decimation0 0"=w371, "LIA Host Interface in"=w372) -> ("error out"=w373:errorcluster, "LIA Host Interface out"=w374:refnum<class "LIA Host Interface.lvclass">)  [unwired: 4 in]
            n139 = call-dynamic "Start Lock-In Channel.vi"("instance"=0 ("index"), "error in"=w373, "config"=w375, "lia host in"=w374) -> ("error out"=w367:errorcluster, "lia host out"=w380:refnum<class "LIA Host Interface.lvclass">)  [unwired: 6 in]
            n140 = flat-sequence {
              tunnel: [w382] -> w368
              tunnel: w367 -> [w382]
              frame #0 {
                n141 = local write "restart averaging  lia"(FALSE ("restart averaging  lia")) -> ()
              }
            }
          }
        }
      }
      frame True {
      }
    }
    n142 = Or(x=w118, y=w119) -> (x .or. y?=w129:bool)
  }
  n143 = Send Notification(notification=TRUE, notifier=w44) -> (notifier out=w42:refnum<notifier>)  [unwired: 1 in, 1 out]
  n144 = Send Notification(notification=TRUE, notifier=w47) -> (notifier out=w43:refnum<notifier>)  [unwired: 1 in, 1 out]
  n145 = flat-sequence {
    tunnel: w43 -> [w390]
    tunnel: w42 -> [_]
    frame #0 {
      n146 = Release Notifier(notifier=w390) -> ()  [unwired: 2 in, 3 out]
    }
  }
  n147 = Merge Errors(w40, w41) -> (w39:errorcluster)
  n148 = call-dynamic "Close.vi"("error in"=w39, "lia host in"=w50) -> ("error out"=w24:errorcluster)  [unwired: 8 in, 1 out]
  n149 = call <vilib>:"Simple Error Handler.vi"("error in (no error)"=w24) -> ()  [unwired: 4 in, 5 out]
